vi "Transport.vi"(4 "Async Elements":refnum<class "Async Elements.lvclass">, 6 "VI Ref":refnum<vi>, 7 "Actor in":refnum<class "Actor.lvclass">, 10 "Refs":refnum<class "Refs.lvclass">) -> (0 "Error out":errorcluster, 5 "Actor out":refnum<class "Actor.lvclass">)   [LabVIEW 2025, in "jettl.lvlib" / "Notifier Transport.lvlib"]
uses:
  Notifier Transport.lvlib
  jettl.lvlib
  Actor/Actor.lvclass
  Refs/Refs.lvclass
  Async Elements/Async Elements.lvclass
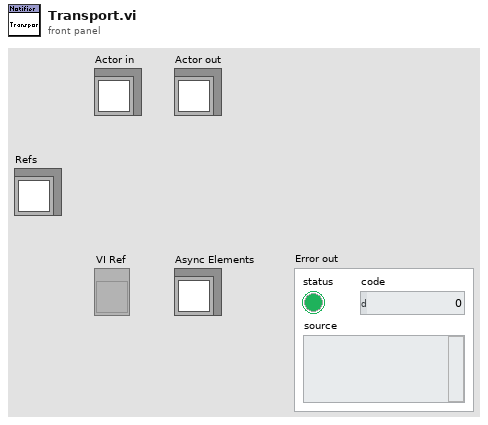
[diagram p1: front panel]
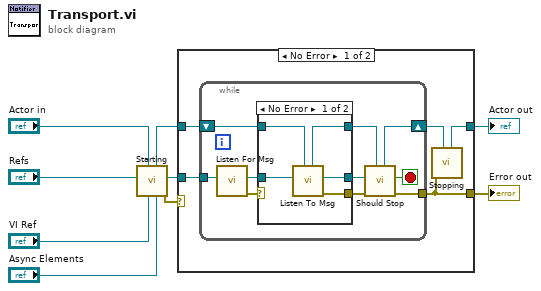
[diagram p0: block diagram]
diagram:
  n1 = call "Starting.vi"("Async Elements"="Async Elements", "VI Ref"="VI Ref", "Actor in"="Actor in", "Refs"="Refs") -> ("Error out"=w5:errorcluster, "Address"=w2:refnum<data-value>, "Actor out"=w6:refnum<class "Actor.lvclass">)  [unwired: 5 in]
  n2 = case shown="No Error" w5 {
    selector: w5 -> [_ w32]
    tunnel: [w12 w33] -> w8
    tunnel: w6 -> [w11 w33]
    tunnel: [w14 w32] -> w9
    tunnel: w2 -> [w10 _]
    frame No Error {
      n3 = while {
        shift-right: [w22] -> w13
        shift-left: w11 -> [w20]
        tunnel: [w23] -> w14
        tunnel: w10 -> [w18]
        stop <- w21 stop-if-true
        n4 = call "Listen For Msg.vi"("Address"=w18) -> ("Error out"=w17:errorcluster, "Msg"=w16:refnum<class "Msg.lvclass">)  [unwired: 9 in]
        n5 = case shown="No Error" w17 {
          selector: w17 -> [_ w30]
          tunnel: [w26 w30] -> w24
          tunnel: w20 -> [w29 w31]
          tunnel: [w27 w31] -> w19
          tunnel: w16 -> [w28 _]
          tunnel: [w25 _] -> w15
          frame No Error {
            n6 = call "Listen To Msg.vi"("Actor in"=w29, "Msg"=w28) -> ("Error out"=w26:errorcluster, "Msg Output"=w25:refnum<class "Msg Output.lvclass">, "Actor out"=w27:refnum<class "Actor.lvclass">)  [unwired: 7 in]
          }
          frame Error {
          }
        }
        n7 = call "Should Stop.vi"("Actor in"=w19, "Error in"=w24, "Msg Output"=w15) -> ("Error out"=w23:errorcluster, "Stop"=w21:bool, "Actor out"=w22:refnum<class "Actor.lvclass">)  [unwired: 6 in]
      }
      n8 = call "Stopping.vi"("Actor in"=w13, "Error in"=w14) -> ("Actor out"=w12:refnum<class "Actor.lvclass">)  [unwired: 9 in]
    }
    frame Error {
    }
  }
  "Error out" <- w9
  "Actor out" <- w8
